vi "Realtime_interaction VI.vi"() -> ()   [LabVIEW 2020]
uses:
  <vilib>/FPGAPlugInAG/cRIO-9054/niLvFpga_Open_cRIO-9054.vi
  <vilib>/rvi/interface/common/dynamic/niFpgaDynamicAddResources.vi
  <vilib>/Utility/error.llb/Error Cluster From Error Code.vi
  <vilib>/rvi/errors/niLvFpgaAdjustHostInterfaceError.vi
  <vilib>/FPGAPlugInAG/Dynamic/niLvFpga_Close_Dynamic.vi
  <vilib>/rvi/interface/nirviOpenFPGA/nirviOpenFPGA.xnode
  FPGA Bitfiles/modifiedtestproj_FPGATarget_FPGAcontrolledVI_2pmID5UxXW8.lvbitx
  FPGA_controlled VI.vi
  <vilib>/rvi/interface/nirviReadWriteControl/nirviReadWriteControl.xnode
  <vilib>/rvi/interface/nirviCloseFPGA/nirviCloseFPGA.xnode
  NiFpgaLv.dll
  <vilib>/rvi/interface/Simulation/niFpgaSimulationCallBeginRW.vi
panel:
  out "Numeric 2":fxp<+/-,20,5> format="%#_5f"
  in  "stop":bool
  in  "Horizontal Pointer Slide":dbl(slide) scale=0.0..10.0 scale format="%#2_3g"
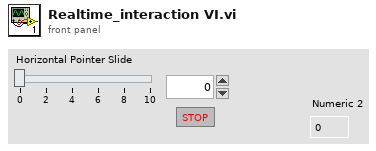
[diagram p1: front panel]
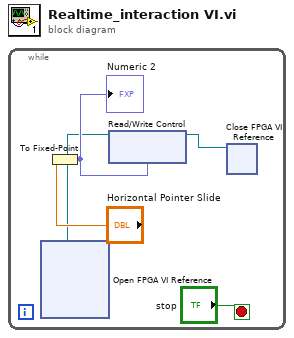
[diagram p0: block diagram]
diagram:
  n1 = while {
    stop <- "stop" stop-if-true
    n2 = xnode "Open FPGA VI Reference"() -> ("FPGA VI Reference Out"=w1:refnum<k20>)  [unwired: 2 in, 1 out]
    n3 = To Fixed-Point(number="Horizontal Pointer Slide") -> (fixed-point=w3:fxp<+/-,20,5>)  [unwired: 1 in]
    "Numeric 2" <- w3
    n4 = xnode "Read/Write Control"("FPGA VI Reference In"=w1, "Mod4/AO0"=w3) -> ("FPGA VI Reference Out"=w2:refnum<k20>)  [unwired: 1 in, 1 out]
    n5 = xnode "Close FPGA VI Reference"("FPGA VI Reference In"=w2) -> ()  [unwired: 1 in, 1 out]
  }
